vi "ExSubOpenCam.vi"(2 "error in (no error)":errorcluster, 3 "Camera Device ID":u32) -> (0 "error out":errorcluster, 1 "Camera Handle":u32)   [LabVIEW 2010]
panel:
  # "ExSubOpenCam:\nThis just opens the camera and nothing else."
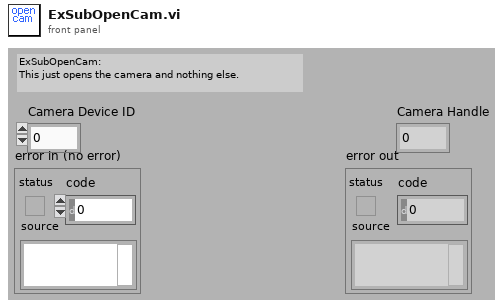
[diagram p1: front panel]
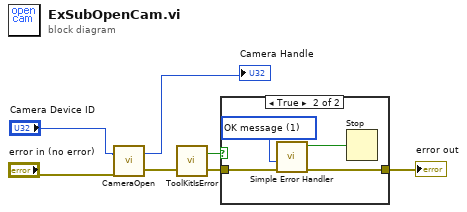
[diagram p0: block diagram]
diagram:
  n1 = call <userlib>:"CameraOpen.vi"("error in"="error in (no error)", "Camera Device ID"="Camera Device ID") -> ("error out"=w6:errorcluster, "Camera Handle"=→"Camera Handle":u32)
  n2 = call <userlib>:"ToolKitIsError.vi"("error in"=w6) -> ("error out"=w4:errorcluster, "Error Flag"=w5:bool)  [unwired: 1 in]
  n3 = case shown="True" w5 {
    tunnel: w4 -> [w8 w12]
    tunnel: [w8 w10] -> w3
    frame False {
    }
    frame True {
      w9 = u16 1 items=["no dialog", "OK message", "continue or stop message"] ("type of dialog (OK msg:1)")
      n4 = call <vilib>:"Simple Error Handler.vi"("type of dialog (OK msg:1)"=w9, "error in (no error)"=w12) -> ("error?"=w11:bool, "error out"=w10:errorcluster)  [unwired: 3 in, 3 out]
      n5 = Stop(stop? (T)=w11) -> ()
    }
  }
  "error out" <- w3
